vi "Do.vi"(8 "error in":errorcluster, 10 "Actor in":refnum<class "Actor.lvclass">, 11 "Update Device Setpoint":refnum<class "Update Device Setpoint.lvclass">) -> (0 "error out":errorcluster, 2 "Actor out":refnum<class "Actor.lvclass">)   [LabVIEW 2014, in "Controller.lvlib" / "Update Device Setpoint.lvclass"]
doc: "(<B>Filename</B>: Actor Framework.lvlib:Message.lvclass:Do.vi)\n\nDefines what a message does when it is received by an actor. Generally, a message instructs an actor to invoke one of its methods. By default, this method does nothing. A child class must override it to define behavior. Create a child class by using the Actor Framework Message Maker dialog box."
uses:
  Update Device Setpoint.lvclass
  <vilib>/ActorFramework/Actor/Actor.lvclass
  Update Device Setpoint.lvclass/Update Device Setpoint.ctl
  Controller.lvclass
  Devices/Configurable Device/Actor/Send New Setpoint MSG/Send New Setpoint.lvclass
  Devices/Configurable Device/Actor/Send New Setpoint MSG/Send New Setpoint.lvclass/Send New Setpoint.ctl
  Controls/eMap.ctl
  <vilib>/ActorFramework/Message Enqueuer/Message Enqueuer.lvclass
  Controller.lvclass/Controller.ctl
  SuperActor/SuperClass.lvclass/SuperClass.ctl
  <vilib>/ActorFramework/Message Enqueuer/Message Enqueuer.lvclass/Message Enqueuer.ctl
  Accessors/Read Enqueuer Map.vi
  SuperActor/Read CVT Session.vi
  SuperActor/Read Log Session.vi
  Devices/Configurable Device/Actor/Send New Setpoint MSG/Write Setpoint.vi
  <vilib>/ActorFramework/Message Priority Queue/Priority Enqueue.vi
  <userlib>/_Session Fwk/Session - Root.lvclass
  reusable/Session APIs/Session Log/System Log.lvclass
  reusable/Session APIs/CVT/CVT.lvclass
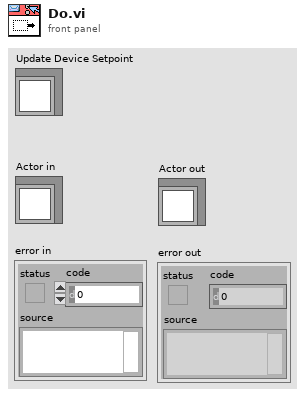
[diagram p1: front panel]
types:
  T1 = typedef "Controller.lvlib/Controller.lvclass/eMap.ctl" = cluster{"Enqueuer":refnum<class "Message Enqueuer.lvclass">, "Active":bool}
  T2 = typedef "Session - Root.lvclass/Session Handle.ctl" = refnum<data-value>
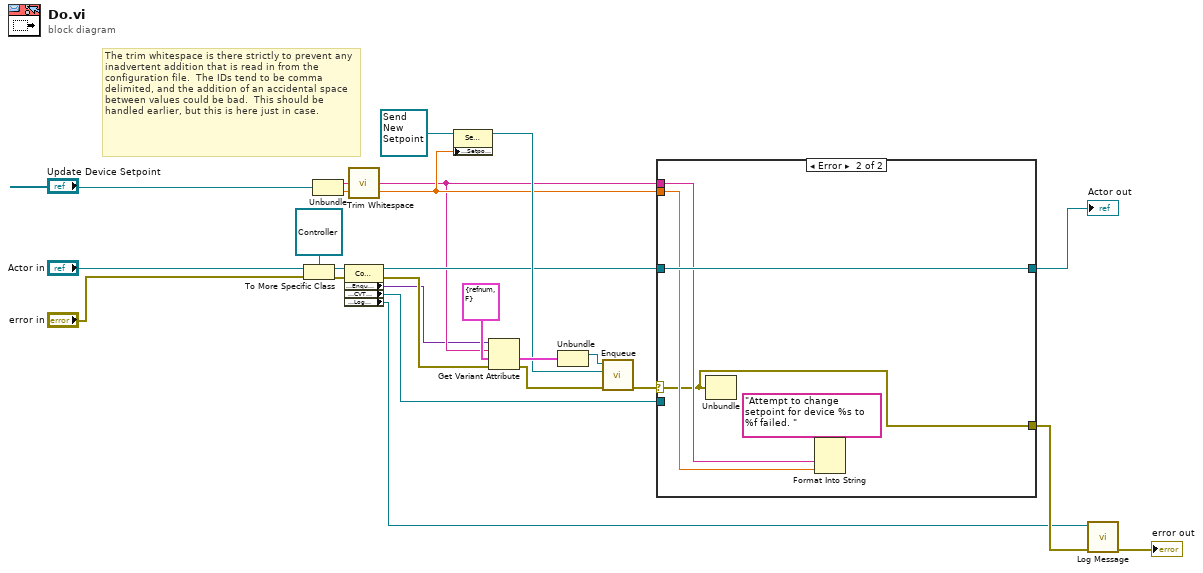
[diagram p0: block diagram]
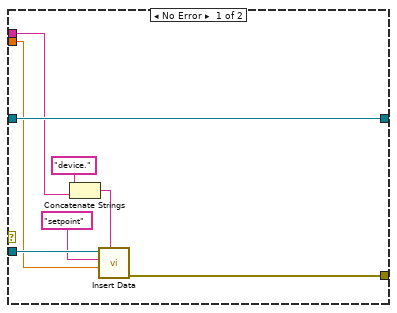
[diagram p2: hidden frame]
diagram:
  # "The trim whitespace is there strictly to prevent any inadvertent addition that is read in from the configuration file.  The IDs tend to be comma delimited, and the addition of an accidental space between values could be bad.  This should be handled earlier, but this is here just in case."
  n1 = To More Specific Class(target class=refnum<class "Controller.lvclass"> refnum ("Controller.lvlib:Controller"), reference="Actor in", error in="error in") -> (specific class reference=w16:refnum<class "Controller.lvclass">, error out=w17:errorcluster)
  n2 = Unbundle("Update Device Setpoint") -> (w8:string, w13:dbl)
  n3 = property class="Controller"(reference=w16, error in=w17) -> (reference out=w14:refnum<class "Controller.lvclass">, error out=w18:errorcluster, "Accessors:Enqueuer Map"=w6:variant, "Accessors:CVT Session"=w10:T2, "Accessors:Log Session"=w9:T2)
  n4 = call <vilib>:"Trim Whitespace.vi"("string"=w8) -> ("trimmed string"=w7:string)  [unwired: 1 in]
  n5 = property class="Send New Setpoint"(reference=refnum<class "Send New Setpoint.lvclass"> refnum ("Device.lvlib:Send New Setpoint"), "Accessors:Setpoint"=w13) -> (reference out=w20:refnum<class "Send New Setpoint.lvclass">)  [unwired: 1 in, 1 out]
  n6 = Get Variant Attribute(Variant=w6, name=w7, default value (empty Variant)=T1 {"Enqueuer"=refnum, "Active"=FALSE} ("eMap"), error in=w18) -> (value=w23:T1, error out=w21:errorcluster)  [unwired: 2 out]
  n7 = Unbundle(w23) -> ("Enqueuer"=w24:refnum<class "Message Enqueuer.lvclass">)  [unwired: 1 out]
  n8 = call <vilib>:"Enqueue.vi"("error in (no error)"=w21, "Message"=w20, "Message Enqueuer in"=w24) -> ("error out"=w11:errorcluster)  [unwired: 7 in, 1 out]
  n9 = case shown="Error" w11 {
    selector: w11 -> [_ w33]
    tunnel: w14 -> [w32 w37]
    tunnel: [w32 w37] -> w2
    tunnel: w7 -> [w28 w35]
    tunnel: w13 -> [w30 w34]
    tunnel: [w29 w33] -> w12
    tunnel: w10 -> [w31 _]
    frame No Error {
      n10 = Concatenate Strings("device." ("string"), w28) -> (w25:string)
      n11 = call "Insert Data.vi"("Group"=w25, "Data"=w30, "tag"="setpoint", "CVT Session In"=w31) -> ("error out"=w29:errorcluster)  [unwired: 6 in, 1 out]
    }
    frame Error {
      n12 = Unbundle(w33) -> ()  [unwired: 3 out]
      n13 = Format Into String(format string="Attempt to change setpoint for device %s to %f failed. ", w35, w34) -> ()  [unwired: 2 in, 2 out]
    }
  }
  "Actor out" <- w2
  n14 = call "Log Message.vi"("error in"=w12, "session in"=w9) -> ("error out"=→"error out":errorcluster)  [unwired: 8 in, 1 out]
